vi "NumIntegrate_Rkf45_impl.vi"(4 "MaxTruncError":dbl, 5 "Func_X_U_Extra":T1, 6 "dT_Remaining":dbl, 7 "PassedData":variant, 8 "InitialH":dbl, 10 "U":T2, 11 "X":T2) -> (0 "Error":bool, 1 "IterationCount":i32, 2 "H":dbl, 3 "NewX":T2)   [LabVIEW 2019, in "Trajectory_Library.lvlib"]
doc: "Implements one loop of RKDP. This takes an initial state, dt guess, and max truncation error, and returns a new x and the dt over which that x was updated. This should be called until there is no dt remaining.\n\nThis is an INTERNAL FUNCTION AND SHOULD NOT BE CALLED DIRECTLY.\n\n\n\nInputs:\n - Func_X_U_Extra -- A strictly typed LabVIEW reference to a function to integrate as a function of matrix X, U, and the extra passed data\n - PassedData -- This is a variant that can be used to pass additional data to the function if needed. The data must be packed into the variant in the specific way expected by the function.\n - X -- The initial value of x.\n - U -- The value u held constant over the integration period.\n - InitialH -- The initial dt guess. This is refined to clamp truncation error to the specified max.\n - dT_Remaining -- How much time is left to integrate over. Used to clamp h.\n - Max TruncError -- The max truncation error acceptable. Usually a small number like 1e-6.\n\nOutputs:\n - New X -- the integration of dx/dt = f(x, u) for dt\n - H -- \n - Iteration count -- How many times this routine looped to achieve the desired error tolerance\n - Error -- If TRUE, an error occured."
uses:
  Trajectory_Library.lvlib
  <vilib>/Analysis/Matrix/NI_Matrix.lvlib
  <vilib>/Analysis/Matrix/Numeric/Multiply/Multiply - RM,R.vi
  <vilib>/Analysis/Matrix/Numeric/Add/Add - RM,RM.vi
  <vilib>/Analysis/Matrix/Datatypes/RealMatrix.ctl
  TypeDef/CALLBACK_FUNC_TYPE.ctl
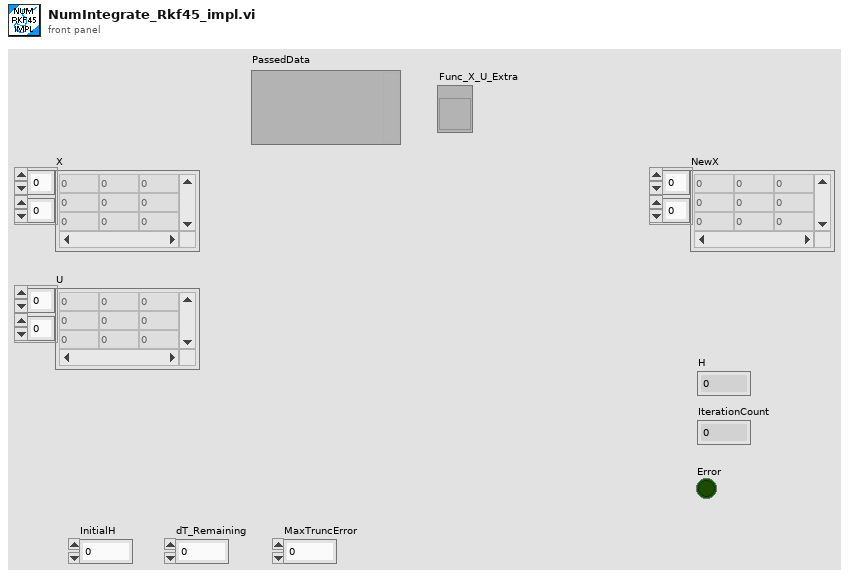
[diagram p1: front panel]
types:
  T1 = typedef "Trajectory_Library.lvlib/CALLBACK_FUNC_TYPE.ctl" = refnum<vi>
  T2 = typedef "NI_Matrix.lvlib/RealMatrix.ctl" = dbl[][]
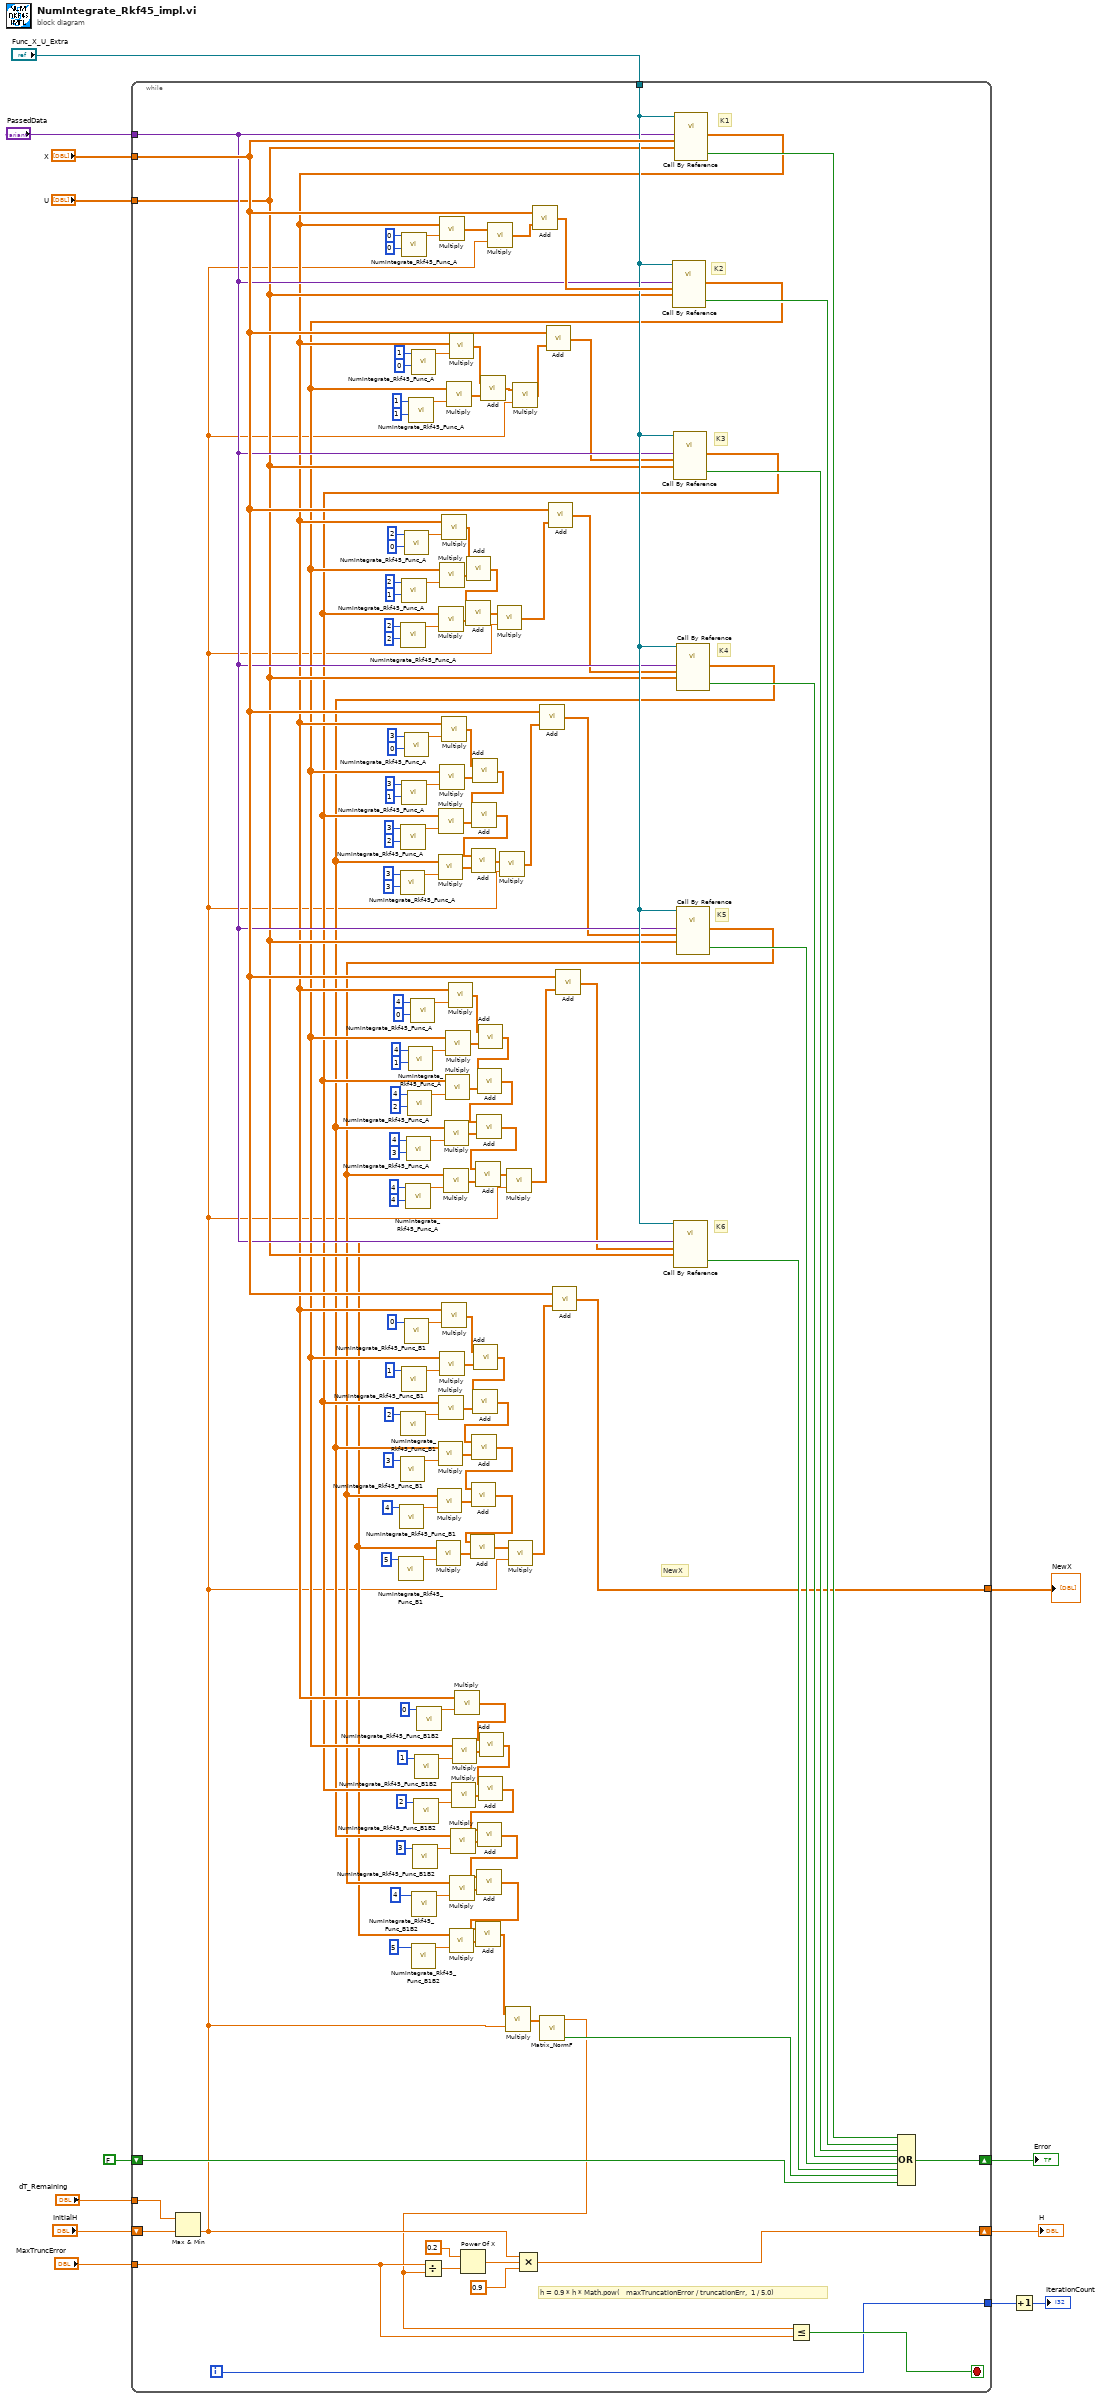
[diagram p0: block diagram]
diagram:
  n1 = while {
    tunnel: "PassedData" -> [w48]
    shift-right: [w64] -> w8
    shift-left: "InitialH" -> [w63]
    tunnel: "X" -> [w58]
    tunnel: "U" -> [w47]
    tunnel: "MaxTruncError" -> [w61]
    tunnel: "dT_Remaining" -> [w62]
    tunnel: [w19] -> w5
    tunnel: [w59] -> w7
    tunnel: "Func_X_U_Extra" -> [w49]
    shift-right: [w50] -> w1
    shift-left: FALSE -> [w57]
    i -> [w59]
    stop <- w60 stop-if-true
    # "K6"
    # "K5"
    # "K4"
    # "K3"
    # "K2"
    # "K1"
    # "h = 0.9 * h * Math.pow(   maxTruncationError / truncationErr,  1 / 5.0)"
    # "NewX"
    n2 = Max & Min(x=w62, y=w63) -> (min(x,y)=w18:dbl)  [unwired: 1 out]
    n3 = call "NumIntegrate_Rkf45_Func_B1.vi"("Index"=5 ("Row")) -> ("RKF45_B1"=w94:dbl)  [unwired: 10 in]
    n4 = call "NumIntegrate_Rkf45_Func_B1.vi"("Index"=4 ("Row")) -> ("RKF45_B1"=w98:dbl)  [unwired: 10 in]
    n5 = call "NumIntegrate_Rkf45_Func_A.vi"("Col"=3, "Row"=3) -> ("RKF45_A"=w138:dbl)  [unwired: 9 in]
    n6 = call "NumIntegrate_Rkf45_Func_B1.vi"("Index"=3 ("Row")) -> ("RKF45_B1"=w102:dbl)  [unwired: 10 in]
    n7 = call "NumIntegrate_Rkf45_Func_A.vi"("Col"=2, "Row"=2) -> ("RKF45_A"=w155:dbl)  [unwired: 9 in]
    n8 = call "NumIntegrate_Rkf45_Func_A.vi"("Col"=2, "Row"=3) -> ("RKF45_A"=w143:dbl)  [unwired: 9 in]
    n9 = call "NumIntegrate_Rkf45_Func_B1.vi"("Index"=2 ("Row")) -> ("RKF45_B1"=w106:dbl)  [unwired: 10 in]
    n10 = call "NumIntegrate_Rkf45_Func_A.vi"("Col"=0, "Row"=0) -> ("RKF45_A"=w173:dbl)  [unwired: 9 in]
    n11 = call "NumIntegrate_Rkf45_Func_A.vi"("Col"=1, "Row"=2) -> ("RKF45_A"=w159:dbl)  [unwired: 9 in]
    n12 = call "NumIntegrate_Rkf45_Func_A.vi"("Col"=1, "Row"=3) -> ("RKF45_A"=w147:dbl)  [unwired: 9 in]
    n13 = call "NumIntegrate_Rkf45_Func_B1.vi"("Index"=1 ("Row")) -> ("RKF45_B1"=w109:dbl)  [unwired: 10 in]
    n14 = call "NumIntegrate_Rkf45_Func_A.vi"("Col"=0, "Row"=2) -> ("RKF45_A"=w162:dbl)  [unwired: 9 in]
    n15 = call "NumIntegrate_Rkf45_Func_A.vi"("Col"=0, "Row"=3) -> ("RKF45_A"=w150:dbl)  [unwired: 9 in]
    n16 = call "NumIntegrate_Rkf45_Func_B1.vi"("Index"=0 ("Row")) -> ("RKF45_B1"=w111:dbl)  [unwired: 10 in]
    n17 = call "NumIntegrate_Rkf45_Func_A.vi"("Col"=4, "Row"=4) -> ("RKF45_A"=w116:dbl)  [unwired: 9 in]
    n18 = call "NumIntegrate_Rkf45_Func_A.vi"("Col"=3, "Row"=4) -> ("RKF45_A"=w121:dbl)  [unwired: 9 in]
    n19 = call "NumIntegrate_Rkf45_Func_A.vi"("Col"=2, "Row"=4) -> ("RKF45_A"=w126:dbl)  [unwired: 9 in]
    n20 = call "NumIntegrate_Rkf45_Func_A.vi"("Col"=1, "Row"=4) -> ("RKF45_A"=w130:dbl)  [unwired: 9 in]
    n21 = call "NumIntegrate_Rkf45_Func_A.vi"("Col"=1, "Row"=1) -> ("RKF45_A"=w166:dbl)  [unwired: 9 in]
    n22 = call "NumIntegrate_Rkf45_Func_A.vi"("Col"=0, "Row"=4) -> ("RKF45_A"=w133:dbl)  [unwired: 9 in]
    n23 = call "NumIntegrate_Rkf45_Func_A.vi"("Col"=0, "Row"=1) -> ("RKF45_A"=w169:dbl)  [unwired: 9 in]
    n24 = call "NumIntegrate_Rkf45_Func_B1B2.vi"("Index"=5 ("Row")) -> ("RKF45_B1-B2"=w73:dbl)  [unwired: 10 in]
    n25 = call "NumIntegrate_Rkf45_Func_B1B2.vi"("Index"=4 ("Row")) -> ("RKF45_B1-B2"=w77:dbl)  [unwired: 10 in]
    n26 = call "NumIntegrate_Rkf45_Func_B1B2.vi"("Index"=3 ("Row")) -> ("RKF45_B1-B2"=w81:dbl)  [unwired: 10 in]
    n27 = call "NumIntegrate_Rkf45_Func_B1B2.vi"("Index"=2 ("Row")) -> ("RKF45_B1-B2"=w85:dbl)  [unwired: 10 in]
    n28 = call "NumIntegrate_Rkf45_Func_B1B2.vi"("Index"=1 ("Row")) -> ("RKF45_B1-B2"=w88:dbl)  [unwired: 10 in]
    n29 = call "NumIntegrate_Rkf45_Func_B1B2.vi"("Index"=0 ("Row")) -> ("RKF45_B1-B2"=w90:dbl)  [unwired: 10 in]
    n30 = call-by-ref "?"(reference=w49, "U"=w47, "X"=w58, "Variant"=w48) -> ("Error"=w51:bool, "NewX"=w46:T2)  [unwired: 8 in, 2 out]
    n31 = call-poly <vilib>:"Multiply.vi"("Real Scalar c"=w173, "Real Matrix A"=w46) -> ("A * c"=w40:T2)
    n32 = call-poly <vilib>:"Multiply.vi"("Real Scalar c"=w162, "Real Matrix A"=w46) -> ("A * c"=w34:T2)
    n33 = call-poly <vilib>:"Multiply.vi"("Real Scalar c"=w150, "Real Matrix A"=w46) -> ("A * c"=w30:T2)
    n34 = call-poly <vilib>:"Multiply.vi"("Real Scalar c"=w111, "Real Matrix A"=w46) -> ("A * c"=w22:T2)
    n35 = call-poly <vilib>:"Multiply.vi"("Real Scalar c"=w133, "Real Matrix A"=w46) -> ("A * c"=w26:T2)
    n36 = call-poly <vilib>:"Multiply.vi"("Real Scalar c"=w169, "Real Matrix A"=w46) -> ("A * c"=w38:T2)
    n37 = call-poly <vilib>:"Multiply.vi"("Real Scalar c"=w90, "Real Matrix A"=w46) -> ("A * c"=w69:T2)
    n38 = call-poly <vilib>:"Multiply.vi"("Real Scalar c"=w18, "Real Matrix A"=w40) -> ("A * c"=w39:T2)
    n39 = call-poly <vilib>:"Add.vi"("Real Matrix B"=w39, "Real Matrix A"=w58) -> ("A + B"=w172:T2)
    n40 = call-by-ref "?"(reference=w49, "U"=w47, "X"=w172, "Variant"=w48) -> ("Error"=w52:bool, "NewX"=w45:T2)  [unwired: 8 in, 2 out]
    n41 = call-poly <vilib>:"Multiply.vi"("Real Scalar c"=w159, "Real Matrix A"=w45) -> ("A * c"=w158:T2)
    n42 = call-poly <vilib>:"Multiply.vi"("Real Scalar c"=w147, "Real Matrix A"=w45) -> ("A * c"=w146:T2)
    n43 = call-poly <vilib>:"Multiply.vi"("Real Scalar c"=w109, "Real Matrix A"=w45) -> ("A * c"=w108:T2)
    n44 = call-poly <vilib>:"Multiply.vi"("Real Scalar c"=w130, "Real Matrix A"=w45) -> ("A * c"=w129:T2)
    n45 = call-poly <vilib>:"Multiply.vi"("Real Scalar c"=w166, "Real Matrix A"=w45) -> ("A * c"=w165:T2)
    n46 = call-poly <vilib>:"Multiply.vi"("Real Scalar c"=w88, "Real Matrix A"=w45) -> ("A * c"=w87:T2)
    n47 = call-poly <vilib>:"Add.vi"("Real Matrix B"=w158, "Real Matrix A"=w34) -> ("A + B"=w151:T2)
    n48 = call-poly <vilib>:"Add.vi"("Real Matrix B"=w146, "Real Matrix A"=w30) -> ("A + B"=w139:T2)
    n49 = call-poly <vilib>:"Add.vi"("Real Matrix B"=w108, "Real Matrix A"=w22) -> ("A + B"=w103:T2)
    n50 = call-poly <vilib>:"Add.vi"("Real Matrix B"=w129, "Real Matrix A"=w26) -> ("A + B"=w122:T2)
    n51 = call-poly <vilib>:"Add.vi"("Real Matrix B"=w87, "Real Matrix A"=w69) -> ("A + B"=w82:T2)
    n52 = call-poly <vilib>:"Add.vi"("Real Matrix B"=w165, "Real Matrix A"=w38) -> ("A + B"=w37:T2)
    n53 = call-poly <vilib>:"Multiply.vi"("Real Scalar c"=w18, "Real Matrix A"=w37) -> ("A * c"=w36:T2)
    n54 = call-poly <vilib>:"Add.vi"("Real Matrix B"=w36, "Real Matrix A"=w58) -> ("A + B"=w35:T2)
    n55 = call-by-ref "?"(reference=w49, "U"=w47, "X"=w35, "Variant"=w48) -> ("Error"=w53:bool, "NewX"=w44:T2)  [unwired: 8 in, 2 out]
    n56 = call-poly <vilib>:"Multiply.vi"("Real Scalar c"=w155, "Real Matrix A"=w44) -> ("A * c"=w154:T2)
    n57 = call-poly <vilib>:"Multiply.vi"("Real Scalar c"=w143, "Real Matrix A"=w44) -> ("A * c"=w142:T2)
    n58 = call-poly <vilib>:"Multiply.vi"("Real Scalar c"=w106, "Real Matrix A"=w44) -> ("A * c"=w105:T2)
    n59 = call-poly <vilib>:"Multiply.vi"("Real Scalar c"=w126, "Real Matrix A"=w44) -> ("A * c"=w125:T2)
    n60 = call-poly <vilib>:"Multiply.vi"("Real Scalar c"=w85, "Real Matrix A"=w44) -> ("A * c"=w84:T2)
    n61 = call-poly <vilib>:"Add.vi"("Real Matrix B"=w154, "Real Matrix A"=w151) -> ("A + B"=w33:T2)
    n62 = call-poly <vilib>:"Add.vi"("Real Matrix B"=w142, "Real Matrix A"=w139) -> ("A + B"=w134:T2)
    n63 = call-poly <vilib>:"Add.vi"("Real Matrix B"=w105, "Real Matrix A"=w103) -> ("A + B"=w99:T2)
    n64 = call-poly <vilib>:"Add.vi"("Real Matrix B"=w125, "Real Matrix A"=w122) -> ("A + B"=w117:T2)
    n65 = call-poly <vilib>:"Add.vi"("Real Matrix B"=w84, "Real Matrix A"=w82) -> ("A + B"=w78:T2)
    n66 = call-poly <vilib>:"Multiply.vi"("Real Scalar c"=w18, "Real Matrix A"=w33) -> ("A * c"=w32:T2)
    n67 = call-poly <vilib>:"Add.vi"("Real Matrix B"=w32, "Real Matrix A"=w58) -> ("A + B"=w31:T2)
    n68 = call-by-ref "?"(reference=w49, "U"=w47, "X"=w31, "Variant"=w48) -> ("Error"=w54:bool, "NewX"=w43:T2)  [unwired: 8 in, 2 out]
    n69 = call-poly <vilib>:"Multiply.vi"("Real Scalar c"=w138, "Real Matrix A"=w43) -> ("A * c"=w137:T2)
    n70 = call-poly <vilib>:"Multiply.vi"("Real Scalar c"=w102, "Real Matrix A"=w43) -> ("A * c"=w101:T2)
    n71 = call-poly <vilib>:"Multiply.vi"("Real Scalar c"=w121, "Real Matrix A"=w43) -> ("A * c"=w120:T2)
    n72 = call-poly <vilib>:"Multiply.vi"("Real Scalar c"=w81, "Real Matrix A"=w43) -> ("A * c"=w80:T2)
    n73 = call-poly <vilib>:"Add.vi"("Real Matrix B"=w137, "Real Matrix A"=w134) -> ("A + B"=w29:T2)
    n74 = call-poly <vilib>:"Add.vi"("Real Matrix B"=w101, "Real Matrix A"=w99) -> ("A + B"=w95:T2)
    n75 = call-poly <vilib>:"Add.vi"("Real Matrix B"=w120, "Real Matrix A"=w117) -> ("A + B"=w112:T2)
    n76 = call-poly <vilib>:"Add.vi"("Real Matrix B"=w80, "Real Matrix A"=w78) -> ("A + B"=w74:T2)
    n77 = call-poly <vilib>:"Multiply.vi"("Real Scalar c"=w18, "Real Matrix A"=w29) -> ("A * c"=w28:T2)
    n78 = call-poly <vilib>:"Add.vi"("Real Matrix B"=w28, "Real Matrix A"=w58) -> ("A + B"=w27:T2)
    n79 = call-by-ref "?"(reference=w49, "U"=w47, "X"=w27, "Variant"=w48) -> ("Error"=w55:bool, "NewX"=w42:T2)  [unwired: 8 in, 2 out]
    n80 = call-poly <vilib>:"Multiply.vi"("Real Scalar c"=w98, "Real Matrix A"=w42) -> ("A * c"=w97:T2)
    n81 = call-poly <vilib>:"Multiply.vi"("Real Scalar c"=w116, "Real Matrix A"=w42) -> ("A * c"=w115:T2)
    n82 = call-poly <vilib>:"Multiply.vi"("Real Scalar c"=w77, "Real Matrix A"=w42) -> ("A * c"=w76:T2)
    n83 = call-poly <vilib>:"Add.vi"("Real Matrix B"=w97, "Real Matrix A"=w95) -> ("A + B"=w91:T2)
    n84 = call-poly <vilib>:"Add.vi"("Real Matrix B"=w115, "Real Matrix A"=w112) -> ("A + B"=w25:T2)
    n85 = call-poly <vilib>:"Add.vi"("Real Matrix B"=w76, "Real Matrix A"=w74) -> ("A + B"=w70:T2)
    n86 = call-poly <vilib>:"Multiply.vi"("Real Scalar c"=w18, "Real Matrix A"=w25) -> ("A * c"=w24:T2)
    n87 = call-poly <vilib>:"Add.vi"("Real Matrix B"=w24, "Real Matrix A"=w58) -> ("A + B"=w23:T2)
    n88 = call-by-ref "?"(reference=w49, "U"=w47, "X"=w23, "Variant"=w48) -> ("Error"=w56:bool, "NewX"=w41:T2)  [unwired: 8 in, 2 out]
    n89 = call-poly <vilib>:"Multiply.vi"("Real Scalar c"=w94, "Real Matrix A"=w41) -> ("A * c"=w93:T2)
    n90 = call-poly <vilib>:"Multiply.vi"("Real Scalar c"=w73, "Real Matrix A"=w41) -> ("A * c"=w72:T2)
    n91 = call-poly <vilib>:"Add.vi"("Real Matrix B"=w93, "Real Matrix A"=w91) -> ("A + B"=w21:T2)
    n92 = call-poly <vilib>:"Add.vi"("Real Matrix B"=w72, "Real Matrix A"=w70) -> ("A + B"=w14:T2)
    n93 = call-poly <vilib>:"Multiply.vi"("Real Scalar c"=w18, "Real Matrix A"=w14) -> ("A * c"=w17:T2)
    n94 = call-poly <vilib>:"Multiply.vi"("Real Scalar c"=w18, "Real Matrix A"=w21) -> ("A * c"=w20:T2)
    n95 = call "Matrix_NormF.vi"("input matrix"=w17) -> ("Error"=w16:bool, "normF"=w15:dbl)  [unwired: 9 in]
    n96 = Divide(x=w61, y=w15) -> (x/y=w67:dbl)
    n97 = Power Of X(1:w67, 2:0.2 ("x")) -> (0:w66:dbl)
    n98 = Compound Arithmetic op=MULTIPLY(w18, w66, 0.9 ("value")) -> (w64:dbl)
    n99 = call-poly <vilib>:"Add.vi"("Real Matrix B"=w20, "Real Matrix A"=w58) -> ("A + B"=w19:T2)
    n100 = Less Or Equal?(x=w15, y=w61) -> (x <= y?=w60:bool)
    n101 = Compound Arithmetic op=OR(w51, w52, w53, w54, w55, w56, w16, w57) -> (w50:bool)
  }
  "NewX" <- w5
  "H" <- w8
  "Error" <- w1
  n102 = Increment(x=w7) -> (x+1=→"IterationCount":i32)
